vi "Populate Accessor Trees.vi"(9 "Folder Tree Ref":refnum<vi>, 10 "Class Item Tree Ref":refnum<vi>, 11 "Class":T3 caption="Object") -> (1 "LVClassLibrary":refnum<vi>, 2 "Folder Tree":T1[](array[typedef]), 3 "Type Tree":T4[](array[typedef]))   [LabVIEW 2018, in "LVClassByRef.lvlib"]
uses:
  <resource>/Framework/Providers/LVClassByRef/LVClassByRef.lvlib
  <resource>/Framework/Providers/LVClassByRef/Type Item.ctl
  <resource>/Framework/Providers/LVClassByRef/Tree Item.ctl
  <vilib>/Utility/Data Type/Type Definitions/Data Type.ctl
  <resource>/Framework/Providers/API/ItemRef.ctl
  <resource>/Framework/Providers/LVClassByRef/Folder Item.ctl
  <vilib>/Utility/Data Type/NI_Data Type.lvlib
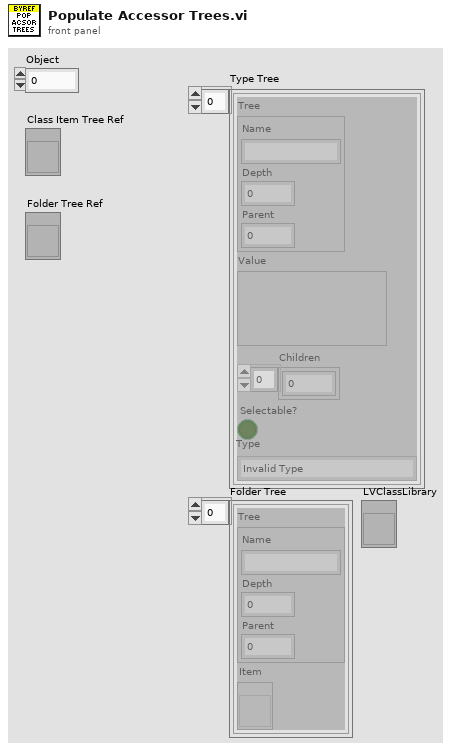
[diagram p1: front panel]
types:
  T1 = typedef "LVClassByRef.lvlib/Folder Item.ctl" = cluster{"Tree":T2, "Item":refnum<vi>}
  T2 = typedef "LVClassByRef.lvlib/Tree Item.ctl" = cluster{"Name":string, "Depth":i32, "Parent":i32}
  T3 = typedef "ItemRef.ctl" = u64
  T4 = typedef "LVClassByRef.lvlib/Type Item.ctl" = cluster{"Tree":T2, "Value":variant, "Children":i32[], "Selectable?":bool, "Type":T5}
  T5 = typedef "NI_Data Type.lvlib/Data Type.ctl" = enum8{"Invalid Type", "Void", "I8", "I16", "I32", "I64", "U8", "U16", "U32", "U64", "Single Float", "Double Float", "Extended Float", "Single Complex", "Double Complex", "Extended Complex", "Enum U8", "Enum U16", "Enum U32", "Enum U64", "Single Float With Unit", "Double Float With Unit", "Extended Float With Unit", "Single Complex with Unit", "Double Complex with Unit", "Extended Complex with Unit", "Boolean", "String", "Path", "Picture", "Tag", "Array", "Cluster", "Variant", "LV Variant", "Waveform", "Timestamp", "Digital Waveform", "Digital Data", "ExpressData", "Refnum", "External Data", "VI", "Poly VI", "LabVIEW Class Instance", "Fixed Point"}
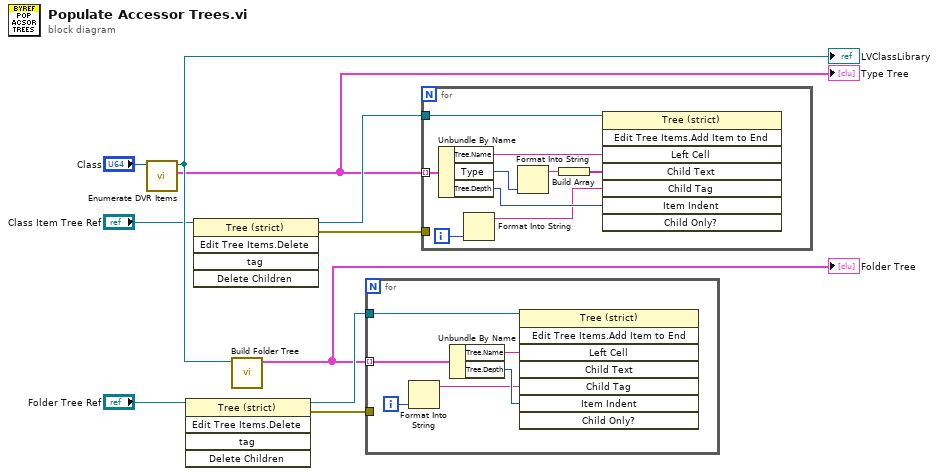
[diagram p0: block diagram]
diagram:
  n1 = call <resource>:"Enumerate DVR Items.vi"("Class"="Class") -> ("Type Tree"=w1:T4[], "LVClassLibrary"=w9:refnum<vi>)  [unwired: 9 in]
  "Type Tree" <- w1
  "LVClassLibrary" <- w9
  n2 = invoke on="Invoke Node" class="Tree (strict)" method="Edit Tree Items.Delete"(reference="Folder Tree Ref") -> (reference out=w4:refnum<vi>, error out=w8:errorcluster)  [unwired: 4 in, 3 out]
  n3 = invoke on="Invoke Node" class="Tree (strict)" method="Edit Tree Items.Delete"(reference="Class Item Tree Ref") -> (reference out=w3:refnum<vi>, error out=w10:errorcluster)  [unwired: 4 in, 3 out]
  n4 = call <resource>:"Build Folder Tree.vi"("Library"=w9) -> ("Folder Tree"=w2:T1[])  [unwired: 10 in]
  "Folder Tree" <- w2
  n5 = for {
    tunnel: w8 -> [_]
    tunnel: w2 -> [w16] mode=indexing
    tunnel: w4 -> [w13]
    i -> [w12]
    n6 = Format Into String(w12) -> (resulting string=w11:string)  [unwired: 3 in, 1 out]
    n7 = Unbundle By Name(w16) -> ("Tree.Name"=w15:string, "Tree.Depth"=w14:i32)
    n8 = invoke on="Invoke Node" class="Tree (strict)" method="Edit Tree Items.Add Item to End"(reference=w13, "Left Cell"=w15, "Child Tag"=w11, "Item Indent"=w14) -> ()  [unwired: 4 in, 8 out]
  }
  n9 = for {
    tunnel: w10 -> [_]
    tunnel: w1 -> [w25] mode=indexing
    tunnel: w3 -> [w19]
    i -> [w18]
    n10 = Unbundle By Name(w25) -> ("Tree.Name"=w24:string, "Type"=w22:T5, "Tree.Depth"=w23:i32)
    n11 = Format Into String(w18) -> (resulting string=w17:string)  [unwired: 3 in, 1 out]
    n12 = Format Into String(w22) -> (resulting string=w21:string)  [unwired: 3 in, 1 out]
    n13 = Build Array(w21) -> (w20:string[])
    n14 = invoke on="Invoke Node" class="Tree (strict)" method="Edit Tree Items.Add Item to End"(reference=w19, "Left Cell"=w24, "Child Text"=w20, "Child Tag"=w17, "Item Indent"=w23) -> ()  [unwired: 3 in, 8 out]
  }
